vi "AB_Get_Default_LVLang.vi"(8 "error in (no error)":errorcluster) -> (0 "error out":errorcluster, 3 "env_language":string)   [LabVIEW 2020]
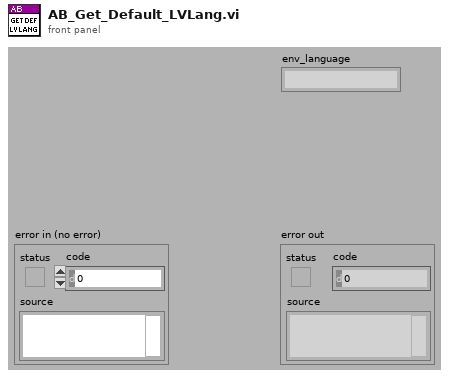
[diagram p1: front panel]
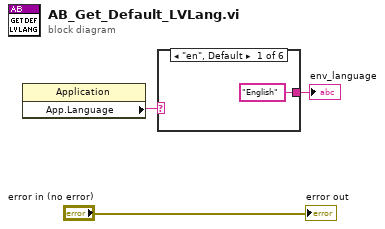
[diagram p0: block diagram]
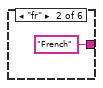
[diagram p2: hidden frame]
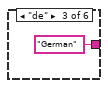
[diagram p3: hidden frame]
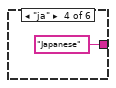
[diagram p4: hidden frame]
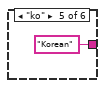
[diagram p5: hidden frame]
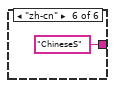
[diagram p6: hidden frame]
diagram:
  n1 = property class="Application"() -> ("App.Language"=w2:string)  [unwired: 2 in, 2 out]
  n2 = case shown="\"en\", Default" w2 {
    tunnel: ["English" ("INI Name") "French" ("INI Name") "German" ("INI Name") "Japanese" ("INI Name") "Korean" ("INI Name") "ChineseS" ("INI Name")] -> w1
    frame "en", Default {
    }
    frame "fr" {
    }
    frame "de" {
    }
    frame "ja" {
    }
    frame "ko" {
    }
    frame "zh-cn" {
    }
  }
  "env_language" <- w1
  "error out" <- "error in (no error)"
